vi "08b_Fronta_zaklady.vi"() -> ()   [LabVIEW 2019]
uses:
  <vilib>/measure/NI_MABase.lvlib
panel:
  in  "Casovani smycky":bool
  out "Prvku ve fronte":i32(slide) scale=0.0..50.0
  in  "Zpozdeni":bool
  out "Producent data":dbl(graph)
  out "Konzument data":dbl(graph)
  out "Konzument Iterace":i32
  out "Producent iterace":i32
  in  "stop":bool
  in  "Amplituda sumu":dbl=0.9999999999999999 format="%.2p"
  in  "Info o vzorkovani":T1={"Vzorkovaci frekvence"=1000.0, "Pocet vzorku v okne"=1000.0} {"Vzorkovaci frekvence" format="%.2p"}
  in  "Faze":dbl format="%.2p"
  in  "Amplituda":dbl=10.0 format="%0.2p"
  in  "Frekvence":dbl=10.0 format="%0.2p"
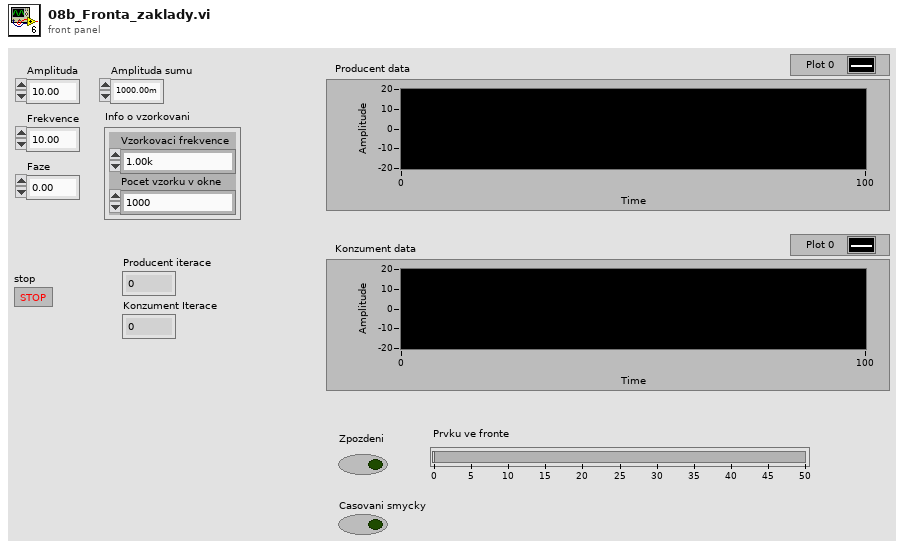
[diagram p1: front panel]
types:
  T1 = cluster{"Vzorkovaci frekvence":dbl, "Pocet vzorku v okne":dbl}
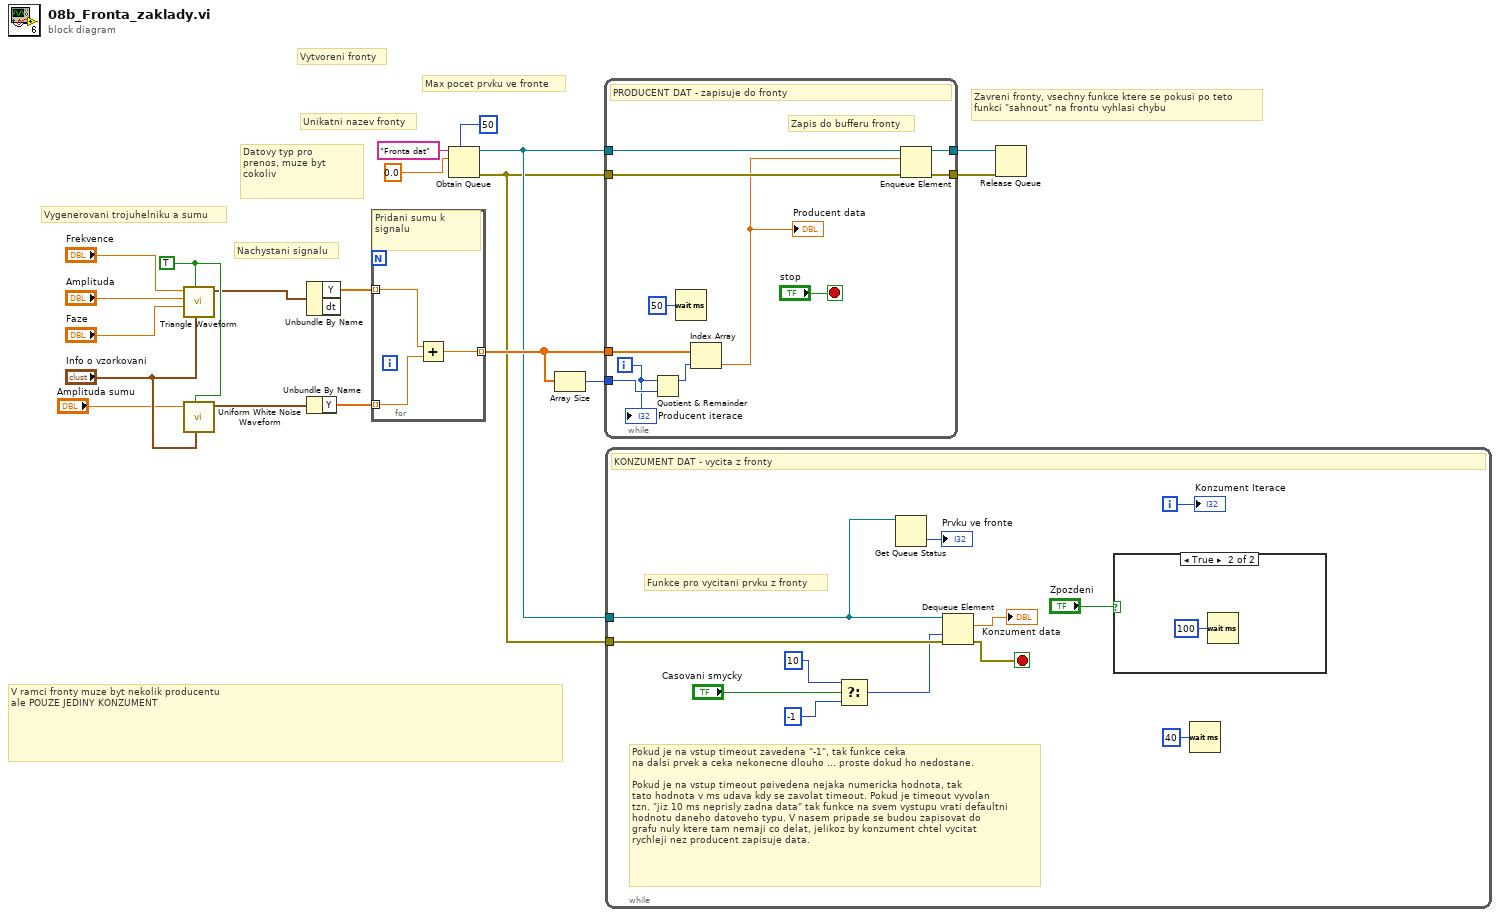
[diagram p0: block diagram]
diagram:
  w14 = TRUE ("reset signal")
  # "V ramci fronty muze byt nekolik producentu\nale POUZE JEDINY KONZUMENT"
  # "Zavreni fronty, vsechny funkce ktere se pokusi po teto \nfunkci \"sahnout\" na frontu vyhlasi chybu"
  # "Datovy typ pro \nprenos, muze byt cokoliv"
  # "Unikatni nazev fronty"
  # "Max pocet prvku ve fronte"
  # "Vytvoreni fronty"
  # "Nachystani signalu"
  # "Vygenerovani trojuhelniku a sumu"
  n1 = call <vilib>:"Triangle Waveform.vi"("sampling info"="Info o vzorkovani", "reset signal"=w14, "phase"="Faze", "amplitude"="Amplituda", "frequency"="Frekvence") -> ("signal out"=w10:waveform(dbl))  [unwired: 5 in, 1 out]
  n2 = call <vilib>:"Uniform White Noise Waveform.vi"("sampling info"="Info o vzorkovani", "reset signal"=w14, "amplitude"="Amplituda sumu") -> ("signal out"=w13:waveform(dbl))  [unwired: 7 in, 1 out]
  n3 = Unbundle By Name(w10) -> ("Y"=w12:dbl[])  [unwired: 1 out]
  n4 = Unbundle By Name(w13) -> ("Y"=w11:dbl[])
  n5 = for {
    tunnel: w12 -> [w21] mode=indexing
    tunnel: w11 -> [w22] mode=indexing
    tunnel: [w20] -> w9 mode=indexing
    # "Pridani sumu k signalu"
    n6 = Add(x=w21, y=w22) -> (x+y=w20:dbl)
  }
  n7 = Obtain Queue(max queue size (-1, unlimited)=50, name (unnamed)="Fronta dat", element data type=0.0) -> (queue out=w4:refnum<queue>, error out=w3:errorcluster)  [unwired: 2 in, 1 out]
  n8 = Array Size(array=w9) -> (size(s)=w8:i32)
  n9 = while {
    tunnel: w9 -> [w31]
    tunnel: w8 -> [w33]
    tunnel: w3 -> [w26]
    tunnel: w4 -> [w27]
    tunnel: [w25] -> w2
    tunnel: [w24] -> w1
    i -> [w32]
    stop <- "stop" stop-if-true
    # "Zapis do bufferu fronty"
    # "PRODUCENT DAT - zapisuje do fronty"
    n10 = Quotient & Remainder(x=w32, y=w33) -> (x-y*floor(x/y)=w30:i32)  [unwired: 1 out]
    n11 = Wait (ms)(milliseconds to wait=u32 50) -> ()  [unwired: 1 out]
    n12 = Index Array(array=w31, index=w30) -> (element=w23:dbl)
    "Producent data" <- w23
    n13 = Enqueue Element(queue=w27, element=w23, error in (no error)=w26) -> (queue out=w25:refnum<queue>, error out=w24:errorcluster)  [unwired: 1 in, 1 out]
    "Producent iterace" <- w32
  }
  n14 = while {
    tunnel: w4 -> [w40]
    tunnel: w3 -> [w45]
    i -> [w43]
    stop <- w44 stop-if-true
    # "Funkce pro vycitani prvku z fronty"
    # "Pokud je na vstup timeout zavedena \"-1\", tak funkce ceka\nna dalsi prvek a ceka nekonecne dlouho ... proste dokud ho nedostane.\n\nPokud je na vstup timeout pøivedena nejaka numericka hodnota, tak\ntato hodnota v ms udava kdy se zavolat timeout. Pokud je timeout vyvolan\ntzn. \"jiz 10 ms neprisly zadna data\" tak funkce na svem vystupu vrati defaultni\nhodnotu daneho datoveho typu. V nasem pripade se budou zapisovat do\ngrafu nuly ktere tam nemaji co delat, jelikoz by konzument chtel vycitat\nrychleji nez producent zapisuje data."
    # "KONZUMENT DAT - vycita z fronty"
    n15 = Select(t=10, s="Casovani smycky", f=-1 ("timeout in ms (-1)")) -> (s? t:f=w36:i32)
    n16 = Get Queue Status(queue=w40) -> (# elements in queue=→"Prvku ve fronte":i32)  [unwired: 2 in, 7 out]
    n17 = Dequeue Element(queue=w40, timeout in ms (-1)=w36, error in (no error)=w45) -> (element=→"Konzument data":dbl, error out=w44:errorcluster)  [unwired: 2 out]
    n18 = case shown="True" "Zpozdeni" {
      frame False {
      }
      frame True {
        n19 = Wait (ms)(milliseconds to wait=u32 100) -> ()  [unwired: 1 out]
      }
    }
    n20 = Wait (ms)(milliseconds to wait=u32 40) -> ()  [unwired: 1 out]
    "Konzument Iterace" <- w43
  }
  n21 = Release Queue(queue=w2, error in (no error)=w1) -> ()  [unwired: 1 in, 3 out]
